vi "Step4.vi"() -> ()   [LabVIEW 2025]
uses:
  <vilib>/Utility/file.llb/Read Delimited Spreadsheet (DBL).vi
  <vilib>/express/express analysis/Spectral/Block/exnSpectralBlock spectral measurements peak poly.vi
  <vilib>/express/express analysis/Spectral/Block/exnSpectralBlock spectral measurements peak DDT.vi
  <vilib>/express/express analysis/Spectral/XNode/ExpressSpectralMeasurementsBlockNode.xnode
  <vilib>/Analysis/NI_AALBase.lvlib
  <vilib>/Analysis/NI_AAL_SigProc.lvlib
panel:
  out "Signal Representation":dbl[](graph)
  out "Amplitudes":dbl[](array[numeric])
  out "Frequency":dbl[](array[numeric])
  out "Fourier Analysis":dynamicdata(graph)
  out "Filtered Signal":dynamicdata(graph)
  out "After Outlier Removal":waveform(dbl)(graph)
  in  "Z Threshold":dbl
  in  "Data File Path":path
  out "Time vs Signal":waveform(dbl)(graph)
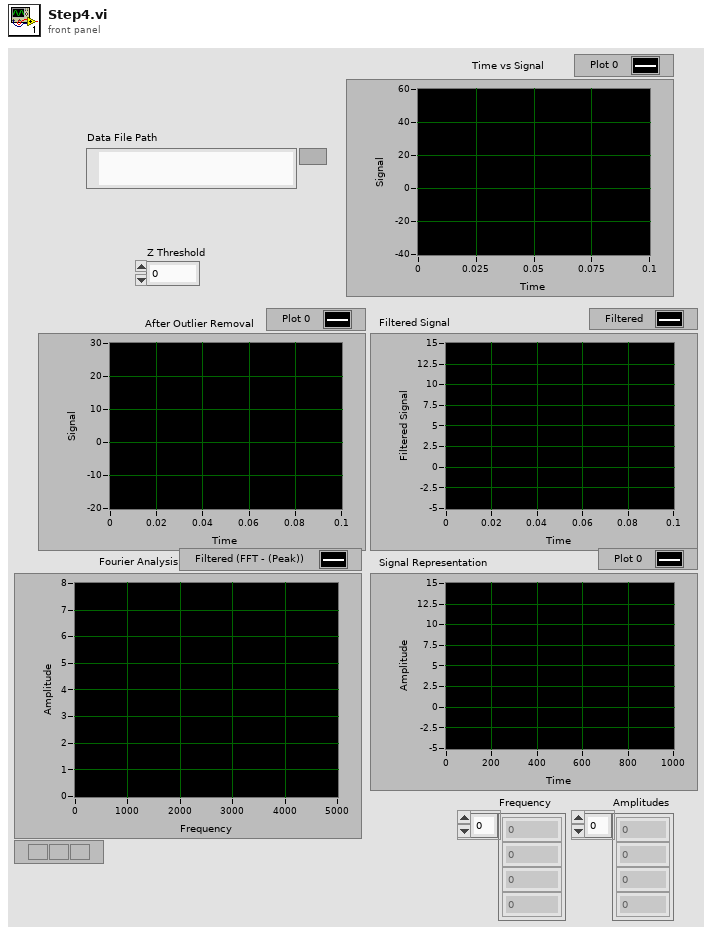
[diagram p1: front panel]
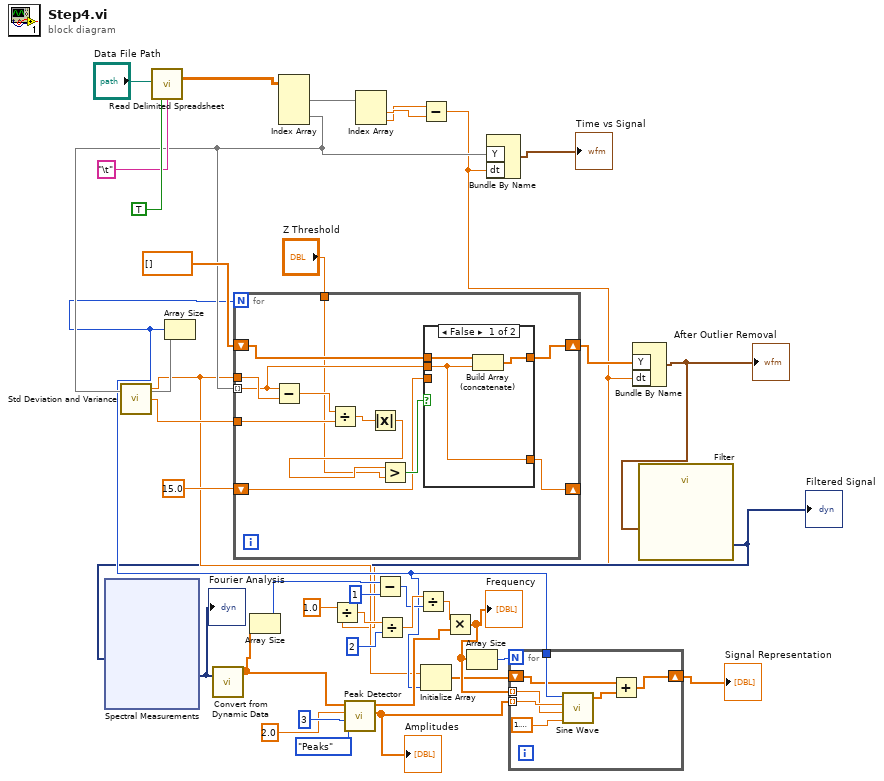
[diagram p0: block diagram]
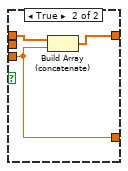
[diagram p2: hidden frame]
diagram:
  n1 = call-poly <vilib>:"Read Delimited Spreadsheet.vi"("file path (dialog if empty)"="Data File Path", "transpose? (F)"=TRUE, "delimiter (\\t)"="\t" ("delimiter (\\t)")) -> ("all rows"=w36:dbl[][])  [unwired: 7 in, 5 out]
  n2 = Index Array(array=w36) -> (element #1=w35:dbl[], element #2=w25:dbl[])  [unwired: 4 in]
  n3 = call <vilib>:"Std Deviation and Variance.vi"("X"=w25) -> ("mean"=w4:dbl, "standard deviation"=w30:dbl)  [unwired: 1 in, 1 out]
  n4 = Array Size(array=w25) -> (size(s)=w6:i32)
  n5 = for {
    N: w6 -> [_]
    shift-right: [w45] -> w27
    tunnel: w30 -> [w49]
    tunnel: w25 -> [w43] mode=indexing
    tunnel: w4 -> [w47]
    tunnel: "Z Threshold" -> [w39]
    shift-left: dbl[] [] -> [w44]
    shift-right: [w41] -> _
    shift-left: 15.0 -> [w42]
    n6 = Subtract(x=w43, y=w47) -> (x-y=w50:dbl)
    n7 = Divide(x=w50, y=w49) -> (x/y=w48:dbl)
    n8 = Absolute Value(x=w48) -> (abs(x)=w40:dbl)
    n9 = Greater?(x=w40, y=w39) -> (0:w46:bool)
    n10 = case shown="False" w46 {
      tunnel: w43 -> [w51 _]
      tunnel: w44 -> [w52 w56]
      tunnel: [w53 w55] -> w45
      tunnel: w42 -> [_ w54]
      tunnel: [w51 w54] -> w41
      frame False {
        n11 = Build Array (concatenate)(w52, w51) -> (w53:dbl[])
      }
      frame True {
        n12 = Build Array (concatenate)(w56, w54) -> (w55:dbl[])
      }
    }
  }
  n13 = Index Array(array=w35) -> (element #1=w34:dbl, element #2=w26:dbl)  [unwired: 2 in]
  n14 = Subtract(x=w26, y=w34) -> (x-y=w1:dbl)
  n15 = Divide(x=1.0, y=w1) -> (x/y=w16:dbl)
  n16 = Divide(x=w16, y=2) -> (x/y=w14:dbl)
  n17 = Initialize Array(w4, w6) -> (w5:dbl[])
  n18 = Bundle By Name("Y"=w25, "dt"=w1) -> (→"Time vs Signal":waveform(dbl))  [unwired: 1 in]
  n19 = Bundle By Name("Y"=w27, "dt"=w1) -> (w24:waveform(dbl))  [unwired: 1 in]
  "After Outlier Removal" <- w24
  n20 = call "Filter"("Signal"=w24) -> ("Filtered Signal"=w3:dynamicdata)  [unwired: 9 in, 1 out]
  "Filtered Signal" <- w3
  n21 = xnode "Spectral Measurements"("Signals"=w3) -> ("FFT - (Peak)"=w20:dynamicdata)  [unwired: 1 in, 2 out]
  "Fourier Analysis" <- w20
  n22 = call "Convert from Dynamic Data"("Dynamic Data Type"=w20) -> ("Array"=w19:dbl[])  [unwired: 3 in]
  n23 = Array Size(array=w19) -> (size(s)=w12:i32)
  n24 = call <vilib>:"Peak Detector.vi"("peaks/valleys"=enum32{"Peaks", "Valleys"}."Peaks", "width"=3, "threshold"=2.0, "X"=w19) -> ("Amplitudes"=w8:dbl[], "Locations"=w11:dbl[])  [unwired: 3 in, 3 out]
  "Amplitudes" <- w8
  n25 = Subtract(x=w12, y=1) -> (x-y=w13:i32)
  n26 = Divide(x=w14, y=w13) -> (x/y=w10:dbl)
  n27 = Multiply(x=w10, y=w11) -> (x*y=w7:dbl[])
  "Frequency" <- w7
  n28 = Array Size(array=w7) -> (size(s)=w9:i32)
  n29 = for {
    N: w9 -> [_]
    tunnel: w8 -> [w62] mode=indexing
    tunnel: w7 -> [w61] mode=indexing
    tunnel: w6 -> [w60]
    shift-right: [w57] -> w2
    shift-left: w5 -> [w58]
    n30 = call <vilib>:"Sine Wave.vi"("samples"=w60, "amplitude"=w62, "frequency"=w61, "phase in"=1.5707963267948966) -> ("sine wave"=w59:dbl[])  [unwired: 1 in, 2 out]
    n31 = Add(x=w58, y=w59) -> (x+y=w57:dbl[])
  }
  "Signal Representation" <- w2
